vi "read hdf dataset.vi"(0 "file":string, 1 "ndims":i32, 2 "shape":i32, 5 "monitor_id":string, 7 "datasetName":string, 9 "data":dbl, 12 "start_index":i32, 13 "strideLength":i32) -> (4 "function return":i32, 6 "monitor_id out":string, 10 "data out":dbl)   [LabVIEW 2019, in "apdm.lvlib"]
doc: "APDM_EXPORT int apdm_read_hdf_dataset(const char *file, char *monitor_id,const char *datasetName, double *data, int ndims, const int *start_index, const int *shape, const int *strideLength);"
uses:
  apdm.lvlib
  Lee Lab/CP FES Walking 2018/Code/Working/LabVIEW/apdm.dll
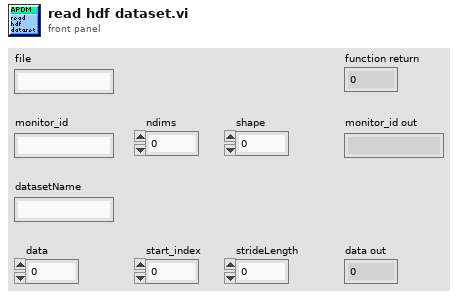
[diagram p1: front panel]
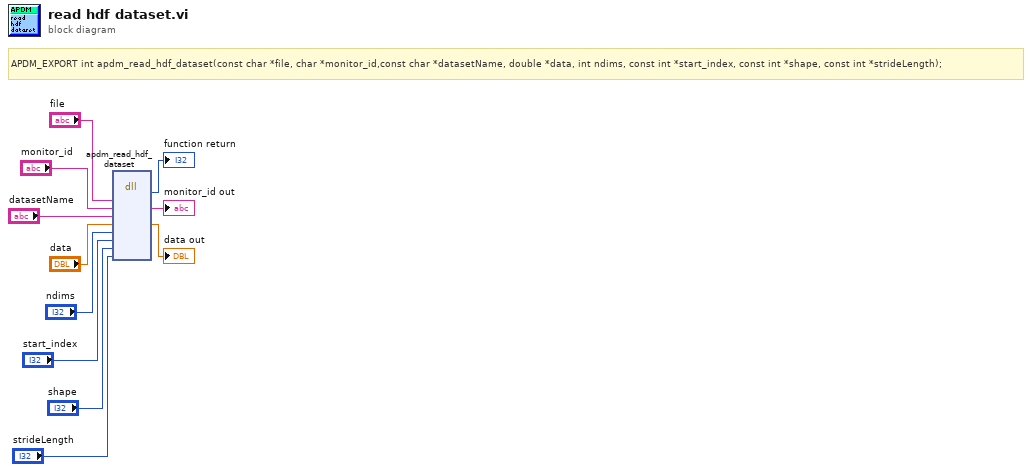
[diagram p0: block diagram]
diagram:
  # "APDM_EXPORT\tint apdm_read_hdf_dataset(const char *file, char *monitor_id,const char *datasetName, double *data, int ndims, const int *start_index, const int *shape, const int *strideLength);"
  n1 = dll-call lib="C:/Users/jfalesi/Dropbox/Lee Lab/CP FES Walking 2018/Code/Working/LabVIEW/apdm.*" fn="apdm_read_hdf_dataset"("file"="file", "monitor_id"="monitor_id", "datasetName"="datasetName", "data"="data", "ndims"="ndims", "start_index"="start_index", "shape"="shape", "strideLength"="strideLength") -> (→"function return":i32, "monitor_id"=→"monitor_id out":string, "data"=→"data out":dbl)  [unwired: 9 in, 2 out]
